vi "Test App Processes are Initialized.vi"(8 "error in (no error)":errorcluster, 11 "Rig Test In":refnum<class "Application Test.lvclass">) -> (0 "error out":errorcluster, 3 "Rig Test Out":refnum<class "Application Test.lvclass">)   [LabVIEW 2020, in "Application Test.lvclass"]
uses:
  Application Test.lvclass
  C:/Program Files (x86)/National Instruments/LabVIEW 2020/vi.lib/Asteme/LUnit/Test Case.lvclass
  Mock Process/Mock Process.lvclass
  C:/Users/anton/Documents/GitHub/Triarc-Framework/source/Framework/Process/Process.lvclass
  Framework/Process/Process.lvclass/Process.ctl
  Framework/Application/Application.lvclass/Application.ctl
  <vilib>/Asteme/LUnit/Test Case.lvclass/Test Case.ctl
  <vilib>/Asteme/LUnit/LUnit Assertion Result.lvclass/LUnit Assertion Result.ctl
  Framework/Process/Protected/SubVIs/Set Context.vi
  Framework/Application/Private/Add Process to Map.vi
  Framework/Process/Protected/Messaging/Enqueue Message.vi
  Framework/Process/Public/Get Lifecycle State.vi
  <vilib>/Asteme/LUnit/Palette/Fail.vi
  <vilib>/Asteme/LUnit/Palette/Pass.vi
  <vilib>/Asteme/LUnit/Set Assertion Type.vi
  Framework/Process/Protected/SubVIs/Get Access Mode.vi
  Framework/Process/Protected/Messaging/Request Message.vi
  Framework/Process/Private/SubVIs/Wait for finish.vi
  Framework/Process/Private/SubVIs/Set Lifecycle State.vi
  <vilib>/AdvancedString/1D String Array to Delimited String.vi
  <vilib>/Utility/error.llb/Clear Errors.vi
  <vilib>/Asteme/LUnit/Add test result.vi
  <vilib>/Asteme/LUnit/LUnit Write Passed.vi
  <vilib>/Asteme/LUnit/LUnit Get Test Case.vi
  <vilib>/Asteme/LUnit/LUnit Write Message.vi
  <vilib>/Asteme/LUnit/LUnit Write Description.vi
  <vilib>/Asteme/LUnit/LUnit Write Assertion Type.vi
  Framework/Process/Private/SubVIs/Enqueue Request Message.vi
  <vilib>/Asteme/LUnit/Read Test Case Name.vi
  Framework/Application/Application.lvclass
  <vilib>/Utility/error.llb/Error Cluster From Error Code.vi
  <vilib>/Asteme/LUnit/Assertion Result/LUnit Get Test Name.vi
  Framework/Process/Private/SubVIs/Wait for Response Message.vi
  Framework/Process/Process.lvclass
  <vilib>/Asteme/LUnit/LUnit Assertion Result.lvclass
  <vilib>/Asteme/LUnit/Test Case.lvclass
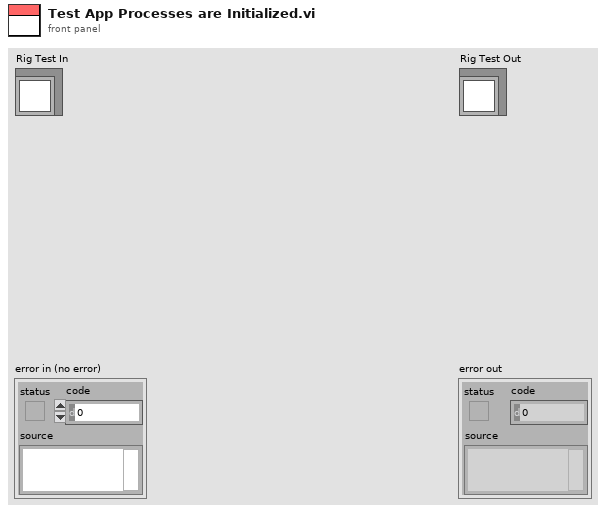
[diagram p1: front panel]
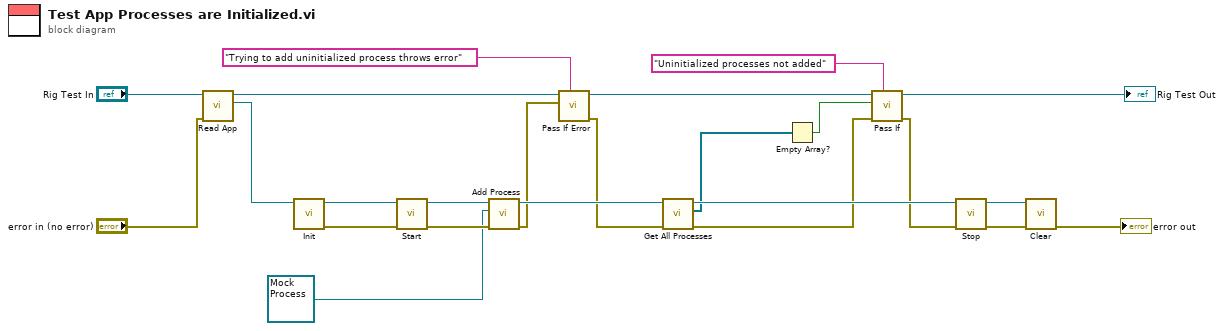
[diagram p0: block diagram]
diagram:
  n1 = call "Read App.vi"("error in (no error)"="error in (no error)", "Application Test In"="Rig Test In") -> ("App out"=w20:refnum<class "Application.lvclass">, "Application Test Out"=w14:refnum<class "Application Test.lvclass">)  [unwired: 7 in, 1 out]
  n2 = call-dynamic "Init.vi"("Process In"=w20) -> ("error out"=w17:errorcluster, "Process Out"=w23:refnum<class "Application.lvclass">)  [unwired: 9 in]
  n3 = call "Start.vi"("error in (no error)"=w17, "Process In"=w23) -> ("error out"=w22:errorcluster, "Process Out"=w16:refnum<class "Application.lvclass">)  [unwired: 8 in]
  n4 = call "Add Process.vi"("error in (no error)"=w22, "Process"=refnum<class "Mock Process.lvclass"> refnum ("Mock Process.lvclass"), "Rig In"=w16) -> ("error out"=w5:errorcluster, "Rig Out"=w19:refnum<class "Application.lvclass">)  [unwired: 7 in]
  n5 = call <vilib>:"Pass If Error.vi"("Description"="Trying to add uninitialized process throws error", "Assert error"=w5, "Test Case In"=w14) -> ("error out"=w4:errorcluster, "Test Case Out"=w6:refnum<class "Application Test.lvclass">)  [unwired: 7 in]
  n6 = call "Get All Processes.vi"("error in (no error)"=w4, "Application In"=w19) -> ("error out"=w13:errorcluster, "App Processes"=w2:refnum<class "Process.lvclass">[], "Application Out"=w15:refnum<class "Application.lvclass">)  [unwired: 7 in]
  n7 = Empty Array?(array=w2) -> (empty?=w3:bool)
  n8 = call <vilib>:"Pass If.vi"("Description"="Uninitialized processes not added", "error in (no error)"=w13, "Pass?"=w3, "Test Case In"=w6) -> ("error out"=w11:errorcluster, "Test Case Out"=→"Rig Test Out":refnum<class "Application Test.lvclass">)  [unwired: 6 in]
  n9 = call "Stop.vi"("error in (no error)"=w11, "Process In"=w15) -> ("error out"=w9:errorcluster, "Process Out"=w21:refnum<class "Application.lvclass">)  [unwired: 7 in, 1 out]
  n10 = call-dynamic "Clear.vi"("error in (no error)"=w9, "Application In"=w21) -> ("error out"=→"error out":errorcluster)  [unwired: 8 in, 1 out]
